vi "Wait is done.vi"(8 "error in":errorcluster, 10 "Axis":i8=1 min=1 max=6 step=1, 11 "Address / Port":i16=1 min=1 max=31 step=1) -> (0 "error out":errorcluster, 2 "Axis out":i8=1 min=1 max=6 step=1, 3 "Address / Port out":i16=1 min=1 max=31 step=1)   [LabVIEW 2014]
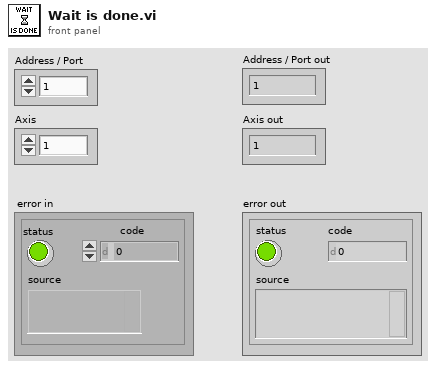
[diagram p1: front panel]
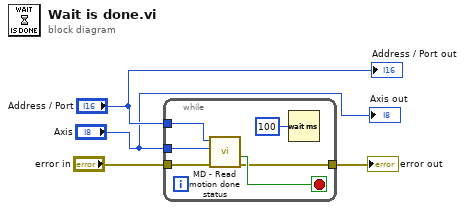
[diagram p0: block diagram]
diagram:
  n1 = while {
    tunnel: [w9] -> w3
    tunnel: "Address / Port" -> [w7]
    tunnel: "Axis" -> [w6]
    tunnel: "error in" -> [w5]
    stop <- w10 stop-if-true
    n2 = call "MD - Read motion done status.vi"("error in"=w5, "Axis"=w6, "Address / Port"=w7) -> ("error out"=w9:errorcluster, "Done"=w10:bool)  [unwired: 5 in, 2 out]
    n3 = Wait (ms)(milliseconds to wait=u32 100) -> ()  [unwired: 1 out]
  }
  "error out" <- w3
  "Address / Port out" <- "Address / Port"
  "Axis out" <- "Axis"
